vi "AutoConvand PID.vi"(8 "Rot SetPoint":dbl, 9 "Y SetPiont":dbl, 10 "X SetPoint":dbl, 11 "Mod State":T1[](array[typedef]) {"Angle"."SIN" format="%13.4f"; "Angle"."COS" format="%13.4f"; "Angle"."VALUE" format="%13.4f"}) -> ()   [LabVIEW 2020]
uses:
  <vilib>/Rock Robotics/WPI/ThirdParty/JAS_Junk/TrajLib/TypeDef/SWERVE_DRIVE_MODULE_STATE.ctl
  <vilib>/Rock Robotics/WPI/ThirdParty/JAS_Junk/TrajLib/TypeDef/ROTATION2D.ctl
  <vilib>/Rock Robotics/WPI/ThirdParty/JAS_Junk/TrajLib/PIDController_AtSetpoint.vi
  <vilib>/Rock Robotics/WPI/ThirdParty/JAS_Junk/TrajLib/PIDController_SetPIDF.vi
  <vilib>/Rock Robotics/WPI/ThirdParty/JAS_Junk/TrajLib/PIDController_SetDerivativeFilter.vi
  <vilib>/Rock Robotics/WPI/ThirdParty/JAS_Junk/TrajLib/PIDController_SetIntegratorRange.vi
  <vilib>/Rock Robotics/WPI/ThirdParty/JAS_Junk/TrajLib/PIDController_SetTolerancePandV.vi
  <vilib>/Rock Robotics/WPI/ThirdParty/JAS_Junk/TrajLib/PIDController_DisableContinousInput.vi
  <vilib>/Rock Robotics/WPI/ThirdParty/JAS_Junk/TrajLib/PIDController_EnableContinousInput.vi
  <vilib>/Rock Robotics/WPI/ThirdParty/JAS_Junk/TrajLib/PIDController_Reset.vi
  <vilib>/Rock Robotics/WPI/ThirdParty/JAS_Junk/TrajLib/PIDController_New.vi
  <vilib>/Rock Robotics/WPI/ThirdParty/JAS_Junk/TrajLib/PIDController_SetOutputLimits.vi
  <vilib>/Rock Robotics/WPI/ThirdParty/JAS_Junk/TrajLib/Rotation2d_GetCos.vi
  <vilib>/Rock Robotics/WPI/ThirdParty/JAS_Junk/TrajLib/Rotation2d_GetSin.vi
  <vilib>/Rock Robotics/WPI/ThirdParty/JAS_Junk/TrajLib/ChassisSpeeds_New.vi
  <vilib>/Rock Robotics/WPI/ThirdParty/JAS_Junk/TrajLib/Conv_Deg_Radians.vi
  <vilib>/Rock Robotics/WPI/ThirdParty/JAS_Junk/TrajLib/Rotation2d_Minus.vi
  <vilib>/Rock Robotics/WPI/ThirdParty/JAS_Junk/TrajLib/Rotation2d_GetRadians.vi
  <vilib>/Rock Robotics/WPI/ThirdParty/JAS_Junk/TrajLib/SwerveModuleState_New.vi
  <vilib>/Rock Robotics/WPI/ThirdParty/JAS_Junk/TrajLib/Rotation2d_RotateBy.vi
  <vilib>/Rock Robotics/WPI/ThirdParty/JAS_Junk/TrajLib/PIDController_NewPeriod.vi
  <vilib>/Rock Robotics/WPI/ThirdParty/JAS_Junk/TrajLib/Rotation2d_UnaryMinus.vi
  <vilib>/Rock Robotics/WPI/ThirdParty/JAS_Junk/TrajLib/Rotation2d_CreateXY.vi
  <vilib>/Rock Robotics/SystemInterfaces/NetworkCommunication/NetComm_UsageReport_report.vi
  <vilib>/Rock Robotics/WPI/ThirdParty/JAS_Junk/TrajLib/Util_CalcDist.vi
  Robot Global Data.vi
  <vilib>/Rock Robotics/WPI/ThirdParty/JAS_Junk/TrajLib/Util_LibraryGlobals.vi
  <vilib>/Rock Robotics/WPI/ThirdParty/JAS_Junk/TrajLib/PIDController_AdvCalculate_FF_Sp_Pv.vi
  <vilib>/Rock Robotics/WPI/ThirdParty/JAS_Junk/TrajLib/Trajectory_Library.lvlib
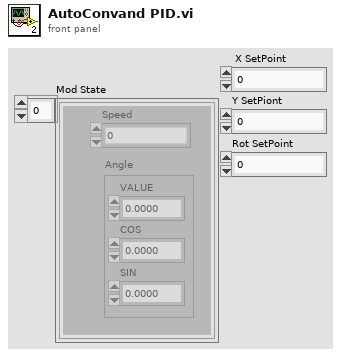
[diagram p1: front panel]
types:
  T1 = typedef "Trajectory_Library.lvlib/SWERVE_DRIVE_MODULE_STATE.ctl" = cluster{"Speed":dbl, "Angle":T2}
  T2 = typedef "Trajectory_Library.lvlib/ROTATION2D.ctl" = cluster{"VALUE":dbl, "COS":dbl, "SIN":dbl}
  T3 = typedef "Trajectory_Library.lvlib/SWERVE_DRIVE_ODOMETRY.ctl" = cluster{"POSE":T4, "GyroOffset":T2, "PreviousAngle":T2, "PrevModulePositions":T6[], "NumModules":i32}
  T4 = typedef "Trajectory_Library.lvlib/POSE2D.ctl" = cluster{"TRANSLATION":T5, "ROTATION":T2}
  T5 = typedef "Trajectory_Library.lvlib/TRANSLATION2D.ctl" = cluster{"X":dbl, "Y":dbl}
  T6 = typedef "Trajectory_Library.lvlib/SWERVE_DRIVE_MODULE_POSITION.ctl" = cluster{"Distance":dbl, "Angle":T2, "P":bool}
  T7 = typedef "Trajectory_Library.lvlib/PID_ADV_LIMITS.ctl" = cluster{"MaxInput":dbl, "MinInput":dbl, "Continuous":bool, "MaxOutput":dbl, "MinOutput":dbl}
  T8 = typedef "Trajectory_Library.lvlib/PID_ADV_TUNING.ctl" = cluster{"Kf":dbl, "Kp":dbl, "Ki":dbl, "Kd":dbl, "MaximumIntegral":dbl, "MinimumIntegral":dbl, "Filter Derivative":bool}
  T9 = typedef "Trajectory_Library.lvlib/SWERVE_DRIVE_KINEMATICS.ctl" = cluster{"NumModules":i32, "InverseKinematics":T10, "ForwardKinematics":T10, "Modules":T5[], "PrevCoR":T5, "SavedModuleStates":T1[]}
  T10 = typedef "NI_Matrix.lvlib/RealMatrix.ctl" = dbl[][]
  T11 = typedef "Trajectory_Library.lvlib/CHASSIS_SPEEDS.ctl" = cluster{"vX":dbl, "vY":dbl, "vOmega":dbl}
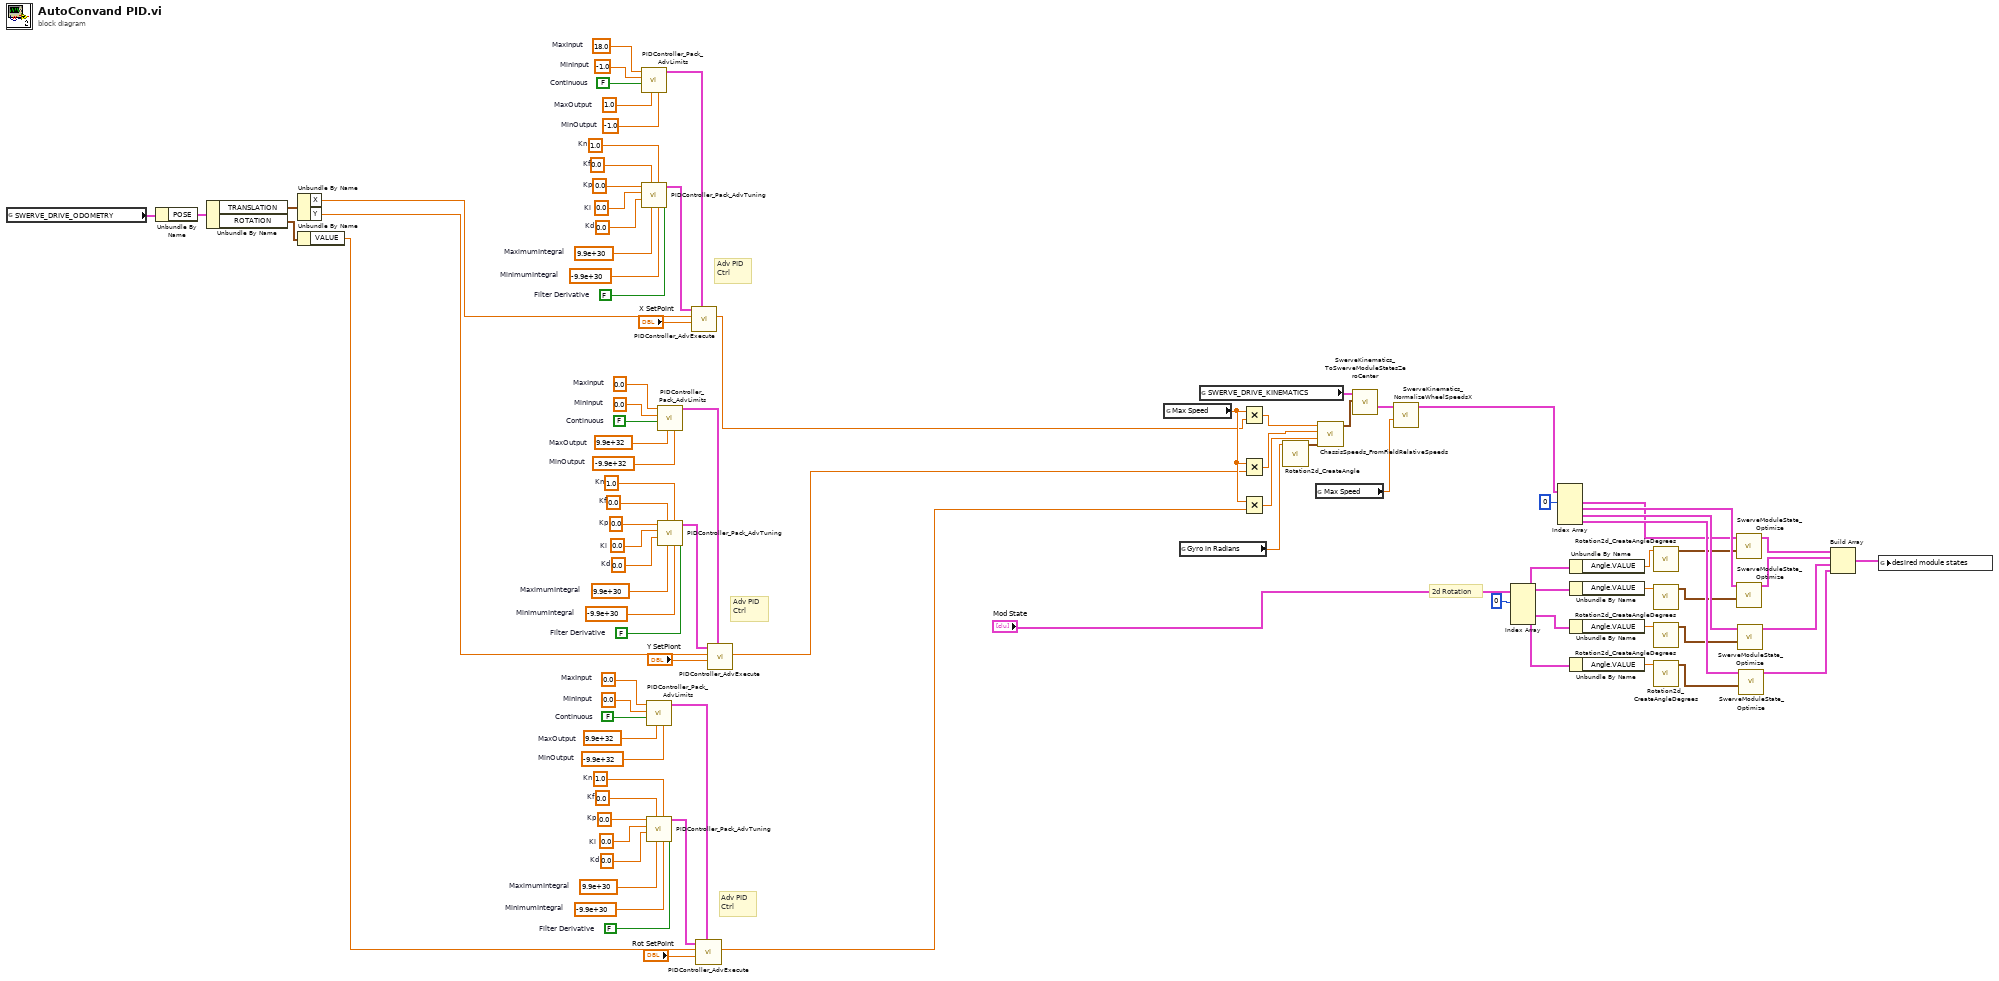
[diagram p0: block diagram]
diagram:
  w28 = 1.0  # Kn
  w27 = 0.0  # Kp
  w26 = 0.0  # Ki
  w25 = 0.0  # Kd
  w24 = 0.0  # Kf
  w23 = 9.9e+30  # MaximumIntegral
  w22 = -9.9e+30  # MinimumIntegral
  w21 = FALSE  # Filter Derivative
  w19 = 0.0  # MinInput
  w18 = FALSE  # Continuous
  w17 = 9.9e+32  # MaxOutput
  w20 = -9.9e+32  # MinOutput
  w16 = 0.0  # MaxInput
  w29 = 1.0  # Kn
  w30 = 0.0  # Kp
  w31 = 0.0  # Ki
  w32 = 0.0  # Kd
  w33 = 0.0  # Kf
  w34 = 9.9e+30  # MaximumIntegral
  w35 = -9.9e+30  # MinimumIntegral
  w36 = FALSE  # Filter Derivative
  w38 = 0.0  # MinInput
  w39 = FALSE  # Continuous
  w40 = 9.9e+32  # MaxOutput
  w37 = -9.9e+32  # MinOutput
  w41 = 0.0  # MaxInput
  w58 = 1.0  # Kn
  w57 = 0.0  # Kp
  w56 = 0.0  # Ki
  w55 = 0.0  # Kd
  w54 = 0.0  # Kf
  w53 = 9.9e+30  # MaximumIntegral
  w52 = -9.9e+30  # MinimumIntegral
  w51 = FALSE  # Filter Derivative
  w49 = -1.0  # MinInput
  w48 = FALSE  # Continuous
  w47 = 1.0  # MaxOutput
  w50 = -1.0  # MinOutput
  w46 = 18.0  # MaxInput
  # "Adv PID\nCtrl"
  # "Adv PID\nCtrl"
  # "Adv PID\nCtrl"
  # "2d Rotation"
  n1 = global read "Robot Global Data.vi" "SWERVE_DRIVE_ODOMETRY"() -> (w10:T3)
  n2 = Unbundle By Name(w10) -> ("POSE"=w9:T4)
  n3 = Unbundle By Name(w9) -> ("TRANSLATION"=w8:T5, "ROTATION"=w5:T2)
  n4 = Unbundle By Name(w8) -> ("X"=w7:dbl, "Y"=w6:dbl)
  n5 = Unbundle By Name(w5) -> ("VALUE"=w4:dbl)
  n6 = call <vilib>:"PIDController_Pack_AdvLimits.vi"("MinOutput"=w50, "MaxOutput"=w47, "Continuous"=w48, "MinInput"=w49, "MaxInput"=w46) -> ("Adv PID Limits"=w44:T7)  [unwired: 6 in]
  n7 = call <vilib>:"PIDController_Pack_AdvTuning.vi"("Filter Derivative"=w51, "MinimumIntegral"=w52, "Kn"=w58, "MaximumIntegral"=w53, "Kf"=w54, "Kd"=w55, "Ki"=w56, "Kp"=w57) -> ("Adv PID Tuning"=w45:T8)  [unwired: 3 in]
  n8 = call <vilib>:"PIDController_Pack_AdvLimits.vi"("MinOutput"=w20, "MaxOutput"=w17, "Continuous"=w18, "MinInput"=w19, "MaxInput"=w16) -> ("Adv PID Limits"=w14:T7)  [unwired: 6 in]
  n9 = call <vilib>:"PIDController_Pack_AdvTuning.vi"("Filter Derivative"=w21, "MinimumIntegral"=w22, "Kn"=w28, "MaximumIntegral"=w23, "Kf"=w24, "Kd"=w25, "Ki"=w26, "Kp"=w27) -> ("Adv PID Tuning"=w15:T8)  [unwired: 3 in]
  n10 = call <vilib>:"PIDController_Pack_AdvLimits.vi"("MinOutput"=w37, "MaxOutput"=w40, "Continuous"=w39, "MinInput"=w38, "MaxInput"=w41) -> ("Adv PID Limits"=w43:T7)  [unwired: 6 in]
  n11 = call <vilib>:"PIDController_Pack_AdvTuning.vi"("Filter Derivative"=w36, "MinimumIntegral"=w35, "Kn"=w29, "MaximumIntegral"=w34, "Kf"=w33, "Kd"=w32, "Ki"=w31, "Kp"=w30) -> ("Adv PID Tuning"=w42:T8)  [unwired: 3 in]
  n12 = call <vilib>:"PIDController_AdvExecute.vi"("Adv PID Limits"=w44, "SP-SetPoint"="X SetPoint", "PV-Measurement"=w7, "Adv PID Tuning"=w45) -> ("CO-ControlOutput"=w13:dbl)  [unwired: 5 in, 2 out]
  n13 = call <vilib>:"PIDController_AdvExecute.vi"("Adv PID Limits"=w14, "SP-SetPoint"="Rot SetPoint", "PV-Measurement"=w4, "Adv PID Tuning"=w15) -> ("CO-ControlOutput"=w11:dbl)  [unwired: 5 in, 2 out]
  n14 = call <vilib>:"PIDController_AdvExecute.vi"("Adv PID Limits"=w43, "SP-SetPoint"="Y SetPiont", "PV-Measurement"=w6, "Adv PID Tuning"=w42) -> ("CO-ControlOutput"=w12:dbl)  [unwired: 5 in, 2 out]
  n15 = global read "Robot Global Data.vi" "Max Speed"() -> (w63:dbl)
  n16 = global read "Robot Global Data.vi" "Gyro in Radians"() -> (w62:dbl)
  n17 = global read "Robot Global Data.vi" "SWERVE_DRIVE_KINEMATICS"() -> (w59:T9)
  n18 = Multiply(x=w63, y=w13) -> (x*y=w93:dbl)
  n19 = Multiply(x=w63, y=w12) -> (x*y=w92:dbl)
  n20 = Multiply(x=w63, y=w11) -> (x*y=w91:dbl)
  n21 = call <vilib>:"Rotation2d_CreateAngle.vi"("Angle"=w62) -> ("ROTATION"=w61:T2)  [unwired: 10 in]
  n22 = global read "Robot Global Data.vi" "Max Speed"() -> (w90:dbl)
  n23 = call <vilib>:"ChassisSpeeds_FromFieldRelativeSpeeds.vi"("RobotAngle"=w61, "Omega"=w91, "vY"=w92, "vX"=w93) -> ("CHASSIS"=w60:T11)  [unwired: 7 in]
  n24 = call <vilib>:"SwerveKinematics_ToSwerveModuleStatesZeroCenter.vi"("ChassisSpeeds"=w60, "in SWERVE_DRIVE_KINEMATICS"=w59) -> ("ModuleStates"=w65:T1[])  [unwired: 8 in, 1 out]
  n25 = call <vilib>:"SwerveKinematics_NormalizeWheelSpeedsX.vi"("AttainableMaxSpeed"=w90, "in WheelStates"=w65) -> ("out WheelStates"=w66:T1[])  [unwired: 9 in]
  n26 = Index Array(array="Mod State", index #1=0 ("index")) -> (element #1=w67:T1, element #2=w74:T1, element #3=w75:T1, element #4=w76:T1)  [unwired: 3 in]
  n27 = Index Array(array=w66, index #1=0 ("index")) -> (element #1=w81:T1, element #2=w82:T1, element #3=w83:T1, element #4=w84:T1)  [unwired: 3 in]
  n28 = Unbundle By Name(w67) -> ("Angle.VALUE"=w70:dbl)
  n29 = Unbundle By Name(w74) -> ("Angle.VALUE"=w71:dbl)
  n30 = Unbundle By Name(w75) -> ("Angle.VALUE"=w72:dbl)
  n31 = Unbundle By Name(w76) -> ("Angle.VALUE"=w73:dbl)
  n32 = call <vilib>:"Rotation2d_CreateAngleDegrees.vi"("Angle_Degrees"=w70) -> ("ROTATION"=w77:T2)  [unwired: 10 in]
  n33 = call <vilib>:"Rotation2d_CreateAngleDegrees.vi"("Angle_Degrees"=w71) -> ("ROTATION"=w78:T2)  [unwired: 10 in]
  n34 = call <vilib>:"Rotation2d_CreateAngleDegrees.vi"("Angle_Degrees"=w72) -> ("ROTATION"=w79:T2)  [unwired: 10 in]
  n35 = call <vilib>:"Rotation2d_CreateAngleDegrees.vi"("Angle_Degrees"=w73) -> ("ROTATION"=w80:T2)  [unwired: 10 in]
  n36 = call <vilib>:"SwerveModuleState_Optimize.vi"("CurrentAngle"=w77, "Desired State"=w81) -> ("out SWERVE_DRIVE_MODULE_STATE"=w85:T1)  [unwired: 9 in]
  n37 = call <vilib>:"SwerveModuleState_Optimize.vi"("CurrentAngle"=w78, "Desired State"=w82) -> ("out SWERVE_DRIVE_MODULE_STATE"=w86:T1)  [unwired: 9 in]
  n38 = call <vilib>:"SwerveModuleState_Optimize.vi"("CurrentAngle"=w79, "Desired State"=w83) -> ("out SWERVE_DRIVE_MODULE_STATE"=w87:T1)  [unwired: 9 in]
  n39 = call <vilib>:"SwerveModuleState_Optimize.vi"("CurrentAngle"=w80, "Desired State"=w84) -> ("out SWERVE_DRIVE_MODULE_STATE"=w88:T1)  [unwired: 9 in]
  n40 = Build Array(w85, w86, w87, w88) -> (w89:T1[])
  n41 = global write "Robot Global Data.vi" "desired module states"(w89) -> ()
